vi "solar_voy_def GUID.vi"() -> (0 "CCSDS_TIME":cluster{"DAY":u16, "MSEC":u32, "USEC":u16}, 1 "TIME_MICROSECONDS":u32, 2 "TIME_SECONDS":u32, 3 "GUID":string)   [LabVIEW 2018]
doc: "This generates a unique GUID and Unix based timestamp. Unix time is offset by midnight 1/1/1970."
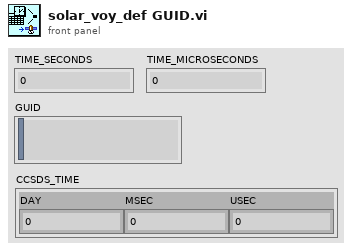
[diagram p1: front panel]
types:
  T1 = typedef "LVDateTimeRec.ctl" = cluster{"fractional second":dbl, "second":i32, "minute":i32, "hour":i32, "day of month":i32, "month":i32, "year":i32, "day of week":i32, "day of year":i32, "DST":i32}
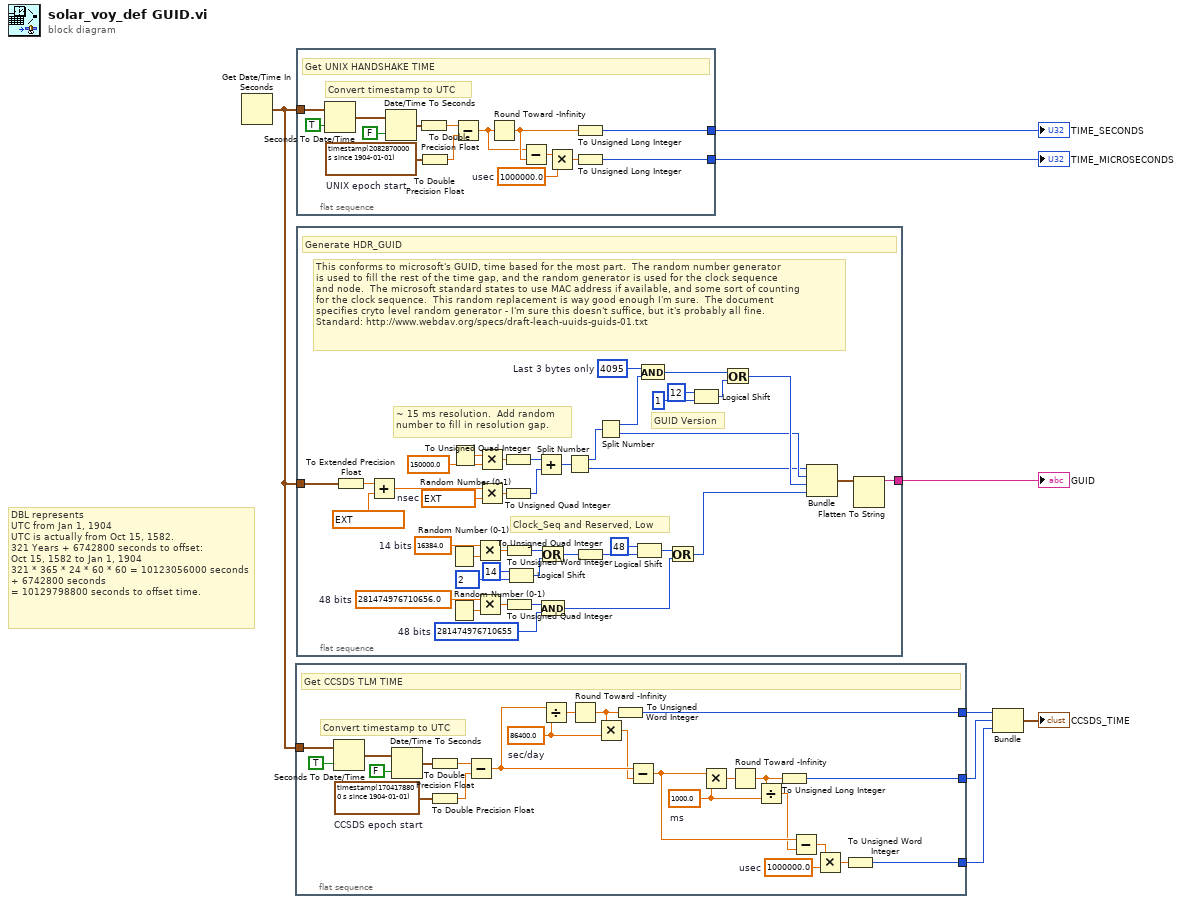
[diagram p0: block diagram]
diagram:
  # "DBL represents\nUTC from Jan 1, 1904\nUTC is actually from Oct 15, 1582.\n321 Years + 6742800 seconds to offset:\nOct 15, 1582 to Jan 1, 1904\n321 * 365 * 24 * 60 * 60 = 10123056000 seconds\n+ 6742800 seconds\n= 10129798800 seconds to offset time."
  n1 = Get Date/Time In Seconds() -> (seconds since 1Jan1904=w2:timestamp)
  n2 = flat-sequence {
    tunnel: [w19] -> w5
    tunnel: [w18] -> w4
    tunnel: [w17] -> w3
    tunnel: w2 -> [w9]
    frame #0 {
      w15 = timestamp(1704178800 s since 1904-01-01)  # CCSDS epoch start
      w20 = 1000000.0  # usec
      w24 = 1000.0  # ms
      w28 = 86400.0  # sec/day
      # "Convert timestamp to UTC"
      # "Get CCSDS TLM TIME"
      n3 = Seconds To Date/Time(time stamp (now)=w9, to UTC (F)=TRUE) -> (date time rec=w12:T1)
      n4 = Date/Time To Seconds(1:FALSE ("is UTC (F)"), 2:w12) -> (0:w11:timestamp)
      n5 = To Double Precision Float(number=w11) -> (double precision float=w10:dbl)
      n6 = To Double Precision Float(number=w15) -> (double precision float=w32:dbl)
      n7 = Subtract(x=w10, y=w32) -> (x-y=w30:dbl)
      n8 = Divide(x=w30, y=w28) -> (x/y=w31:dbl)
      n9 = Round Toward -Infinity(1:w31) -> (0:w29:dbl)
      n10 = Multiply(x=w29, y=w28) -> (x*y=w27:dbl)
      n11 = To Unsigned Word Integer(number=w29) -> (unsigned 16bit integer=w19:u16)
      n12 = Subtract(x=w30, y=w27) -> (x-y=w23:dbl)
      n13 = Multiply(x=w23, y=w24) -> (x*y=w26:dbl)
      n14 = Round Toward -Infinity(1:w26) -> (0:w25:dbl)
      n15 = Divide(x=w25, y=w24) -> (x/y=w22:dbl)
      n16 = To Unsigned Long Integer(number=w25) -> (unsigned 32bit integer=w18:u32)
      n17 = Subtract(x=w23, y=w22) -> (x-y=w21:dbl)
      n18 = Multiply(x=w21, y=w20) -> (x*y=w16:dbl)
      n19 = To Unsigned Word Integer(number=w16) -> (unsigned 16bit integer=w17:u16)
    }
  }
  n20 = flat-sequence {
    tunnel: [w35] -> w8
    tunnel: [w34] -> w7
    tunnel: w2 -> [w33]
    frame #0 {
      w40 = 1000000.0  # usec
      w38 = timestamp(2082870000 s since 1904-01-01)  # UNIX epoch start
      # "Convert timestamp to UTC"
      # "Get UNIX HANDSHAKE TIME"
      n21 = Seconds To Date/Time(time stamp (now)=w33, to UTC (F)=TRUE) -> (date time rec=w46:T1)
      n22 = Date/Time To Seconds(1:FALSE ("is UTC (F)"), 2:w46) -> (0:w47:timestamp)
      n23 = To Double Precision Float(number=w47) -> (double precision float=w36:dbl)
      n24 = To Double Precision Float(number=w38) -> (double precision float=w37:dbl)
      n25 = Subtract(x=w36, y=w37) -> (x-y=w39:dbl)
      n26 = Round Toward -Infinity(1:w39) -> (0:w42:dbl)
      n27 = Subtract(x=w39, y=w42) -> (x-y=w43:dbl)
      n28 = Multiply(x=w43, y=w40) -> (x*y=w41:dbl)
      n29 = To Unsigned Long Integer(number=w42) -> (unsigned 32bit integer=w35:u32)
      n30 = To Unsigned Long Integer(number=w41) -> (unsigned 32bit integer=w34:u32)
    }
  }
  n31 = flat-sequence {
    tunnel: [w52] -> w6
    tunnel: w2 -> [w48]
    frame #0 {
      w50 = ext 10000000.0  # nsec
      w85 = u64 281474976710655  # 48 bits
      w83 = 281474976710656.0  # 48 bits
      w74 = 16384.0  # 14 bits
      w63 = u16 4095  # Last 3 bytes only
      # "Clock_Seq and Reserved, Low"
      # "This conforms to microsoft's GUID, time based for the most part.  The random number generator\nis used to fill the rest of the time gap, and the random generator is used for the clock sequence\nand node.  The microsoft standard states to use MAC address if available, and some sort of counting\nfor the clock sequence.  This random replacement is way good enough I'm sure.  The document\nspecifies cryto level random generator - I'm sure this doesn't suffice, but it's probably all fine.\nStandard: http://www.webdav.org/specs/draft-leach-uuids-guids-01.txt"
      # "GUID Version"
      # "~ 15 ms resolution.  Add random\nnumber to fill in resolution gap."
      # "Generate HDR_GUID"
      n32 = To Extended Precision Float(1:w48) -> (0:w59:ext)
      n33 = Add(x=w59, y=ext 10129798800.0) -> (x+y=w51:ext)
      n34 = Random Number (0-1)() -> (number: 0 to 1=w75:dbl)
      n35 = Random Number (0-1)() -> (number: 0 to 1=w82:dbl)
      n36 = Random Number (0-1)() -> (number: 0 to 1=w68:dbl)
      n37 = Multiply(x=w74, y=w75) -> (x*y=w76:dbl)
      n38 = Multiply(x=w83, y=w82) -> (x*y=w81:dbl)
      n39 = Multiply(x=w68, y=150000.0 ("Count32L")) -> (x*y=w70:dbl)
      n40 = Multiply(x=w51, y=w50) -> (x*y=w49:ext)
      n41 = To Unsigned Quad Integer(1:w70) -> (0:w71:u64)
      n42 = To Unsigned Quad Integer(1:w49) -> (0:w72:u64)
      n43 = To Unsigned Word Integer(number=w76) -> (unsigned 16bit integer=w77:u16)
      n44 = To Unsigned Quad Integer(1:w81) -> (0:w84:u64)
      n45 = Logical Shift(y=u16 14, x=u16 2) -> (x << y=w80:u16)
      n46 = Add(x=w71, y=w72) -> (x+y=w73:u64)
      n47 = Or(x=w77, y=w80) -> (x .or. y?=w54:u16)
      n48 = And(x=w84, y=w85) -> (x .and. y?=w55:u64)
      n49 = Split Number(x=w73) -> (hi(x)=w61:u32, lo(x)=w86:u32)
      n50 = To Unsigned Quad Integer(1:w54) -> (0:w58:u64)
      n51 = Split Number(x=w61) -> (hi(x)=w62:u16, lo(x)=w87:u16)
      n52 = Logical Shift(y=i8 48, x=w58) -> (x << y=w56:u64)
      n53 = And(x=w63, y=w62) -> (x .and. y?=w67:u16)
      n54 = Or(x=w56, y=w55) -> (x .or. y?=w53:u64)
      n55 = Logical Shift(y=u16 12, x=u16 1) -> (x << y=w64:u16)
      n56 = Or(x=w67, y=w64) -> (x .or. y?=w88:u16)
      n57 = Bundle(w86, w87, w88, w53) -> (w89:cluster{u32, u16, u16, u64})  [unwired: 1 in]
      n58 = Flatten To String(anything=w89) -> (data string=w52:string)  [unwired: 3 in, 2 out]
    }
  }
  n59 = Bundle(w5, w4, w3) -> (→"CCSDS_TIME":cluster{u16, u32, u16})  [unwired: 1 out]
  "TIME_SECONDS" <- w8
  "TIME_MICROSECONDS" <- w7
  "GUID" <- w6
